vi "Descanner1_Analog_PMT.vi"(0 "Pix":i32, 1 "scanPix":i32, 2 "delta_p":i32, 3 "Data":dbl[](array[numeric])) -> (5 "2Lines":dbl[][](array[numeric]))   [LabVIEW 2016]
panel:
  out "size(s)":i32[](array[numeric])
  out "Waveform Graph":dbl[](graph)
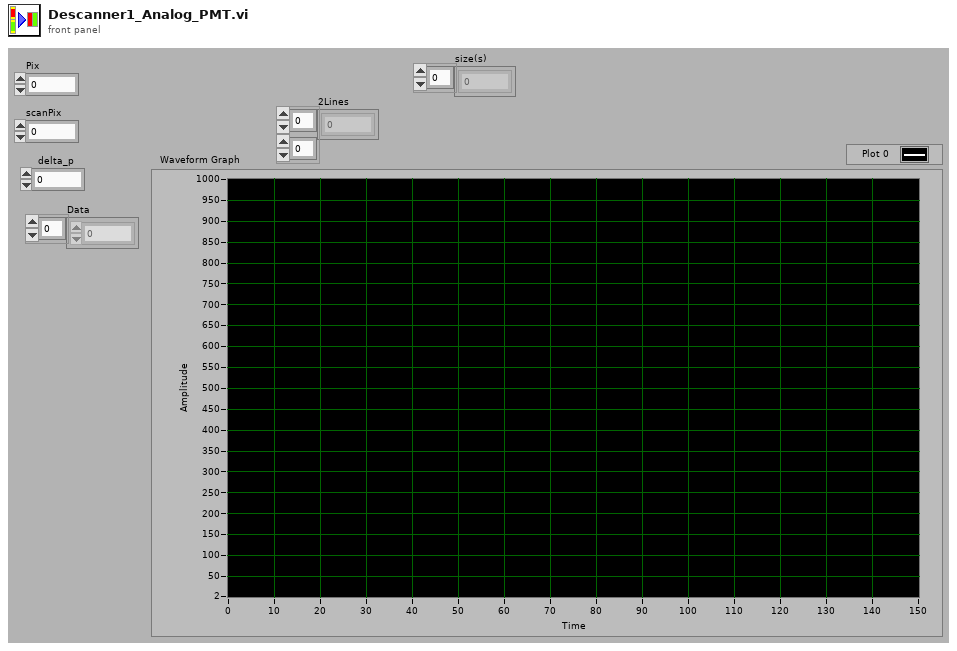
[diagram p1: front panel]
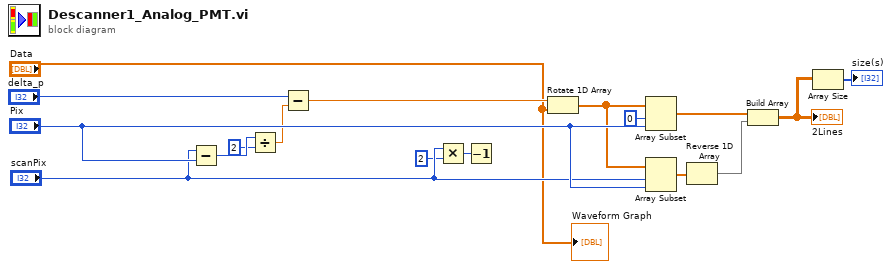
[diagram p0: block diagram]
diagram:
  n1 = Subtract(x="scanPix", y="Pix") -> (x-y=w17:i32)
  n2 = Divide(x=w17, y=2) -> (x/y=w5:dbl)
  n3 = Subtract(x="delta_p", y=w5) -> (x-y=w12:dbl)
  n4 = Multiply(x="scanPix", y=2) -> (x*y=w7:i32)
  n5 = Decrement(x=w7) -> ()  [unwired: 1 out]
  n6 = Rotate 1D Array(1:"Data", 2:w12) -> (0:w4:dbl[])
  n7 = Array Subset(array=w4, index=0, length="Pix") -> (w6:dbl[])
  n8 = Array Subset(array=w4, index="scanPix", length="Pix") -> (w13:dbl[])
  n9 = Reverse 1D Array(array=w13) -> (reversed array=w10:dbl[])
  n10 = Build Array(w6, w10) -> (w3:dbl[][])
  "2Lines" <- w3
  n11 = Array Size(array=w3) -> (size(s)=→"size(s)":i32[])
  "Waveform Graph" <- "Data"
